vi "Set Refnums.vi"   [LabVIEW 2013]
uses:
  <vilib>/Rock Robotics/WPI/DriverStation/WPI_DriverStationRobotMode2.ctl
  Global Refnums.vi
  Robot Global Data.vi
types:
  T1 = typedef "WPI_DriverStationRobotMode2.ctl" = enum16{"Autonomous Disabled", "Autonomous Enabled", "Teleop Disabled", "Teleop Enabled", "Timeout", "Finish", "Test Disabled", "Test Enabled"}
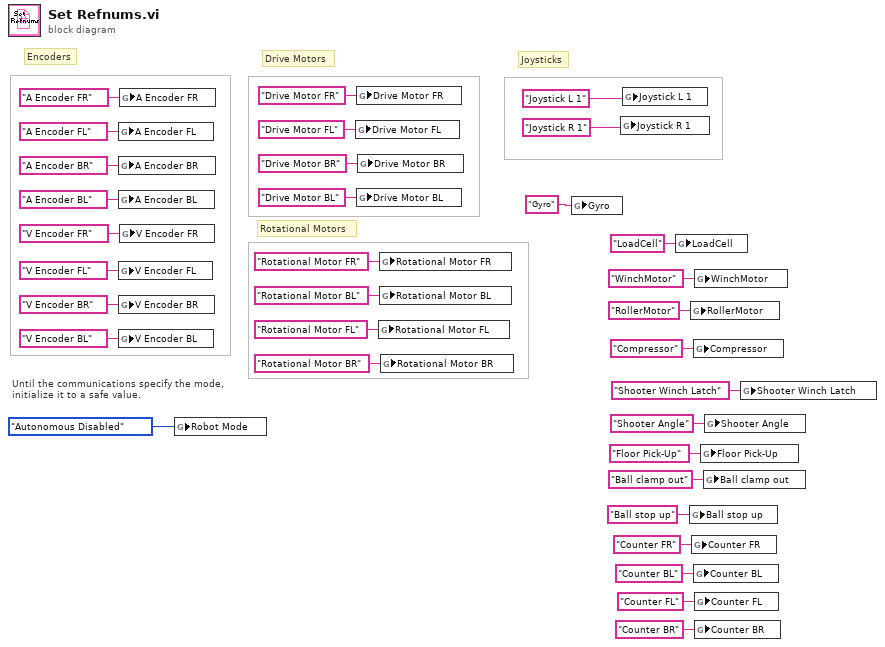
[diagram p0: block diagram]
diagram:
  # "Until the communications specify the mode,\ninitialize it to a safe value."
  # "Joysticks"
  # "Rotational Motors"
  # "Encoders"
  # "Drive Motors"
  n1 = global write "Global Refnums.vi" "A Encoder FL"("A Encoder FL") -> ()
  n2 = global write "Global Refnums.vi" "A Encoder BR"("A Encoder BR") -> ()
  n3 = global write "Global Refnums.vi" "A Encoder BL"("A Encoder BL") -> ()
  n4 = global write "Global Refnums.vi" "V Encoder FL"("V Encoder FL") -> ()
  n5 = global write "Global Refnums.vi" "V Encoder BR"("V Encoder BR") -> ()
  n6 = global write "Global Refnums.vi" "V Encoder BL"("V Encoder BL") -> ()
  n7 = global write "Global Refnums.vi" "A Encoder FR"("A Encoder FR") -> ()
  n8 = global write "Global Refnums.vi" "V Encoder FR"("V Encoder FR") -> ()
  n9 = global write "Robot Global Data.vi" "Robot Mode"(WPI_DriverStationRobotMode2."Autonomous Disabled" ("Robot Mode")) -> ()
  n10 = global write "Global Refnums.vi" "Drive Motor FL"("Drive Motor FL") -> ()
  n11 = global write "Global Refnums.vi" "Drive Motor FR"("Drive Motor FR") -> ()
  n12 = global write "Global Refnums.vi" "Drive Motor BL"("Drive Motor BL") -> ()
  n13 = global write "Global Refnums.vi" "Drive Motor BR"("Drive Motor BR") -> ()
  n14 = global write "Global Refnums.vi" "Rotational Motor FL"("Rotational Motor FL") -> ()
  n15 = global write "Global Refnums.vi" "Rotational Motor FR"("Rotational Motor FR") -> ()
  n16 = global write "Global Refnums.vi" "Rotational Motor BL"("Rotational Motor BL") -> ()
  n17 = global write "Global Refnums.vi" "Rotational Motor BR"("Rotational Motor BR") -> ()
  n18 = global write "Global Refnums.vi" "Gyro"("Gyro") -> ()
  n19 = global write "Global Refnums.vi" "Joystick R 1"("Joystick R 1") -> ()
  n20 = global write "Global Refnums.vi" "Joystick L 1"("Joystick L 1") -> ()
  n21 = global write "Global Refnums.vi" "LoadCell"("LoadCell") -> ()
  n22 = global write "Global Refnums.vi" "Ball stop up"("Ball stop up") -> ()
  n23 = global write "Global Refnums.vi" "RollerMotor"("RollerMotor") -> ()
  n24 = global write "Global Refnums.vi" "Counter FR"("Counter FR") -> ()
  n25 = global write "Global Refnums.vi" "Compressor"("Compressor") -> ()
  n26 = global write "Global Refnums.vi" "Counter BL"("Counter BL") -> ()
  n27 = global write "Global Refnums.vi" "WinchMotor"("WinchMotor") -> ()
  n28 = global write "Global Refnums.vi" "Counter FL"("Counter FL") -> ()
  n29 = global write "Global Refnums.vi" "Counter BR"("Counter BR") -> ()
  n30 = global write "Global Refnums.vi" "Floor Pick-Up"("Floor Pick-Up") -> ()
  n31 = global write "Global Refnums.vi" "Ball clamp out"("Ball clamp out") -> ()
  n32 = global write "Global Refnums.vi" "Shooter Angle"("Shooter Angle") -> ()
  n33 = global write "Global Refnums.vi" "Shooter Winch Latch"("Shooter Winch Latch") -> ()
